vi "Override maxSensorNum (O).vi"(8 "Error In":errorcluster, 10 "Max. number of sensors":u8 max=64, 11 "VISA resource name in":refnum<visa-resource-name>) -> (0 "Error out":errorcluster, 1 "ACK":bool, 2 "L_data":u16, 3 "VISA resource name out":refnum<visa-resource-name>)   [LabVIEW 2015]
uses:
  Ctls/Cmd str.ctl
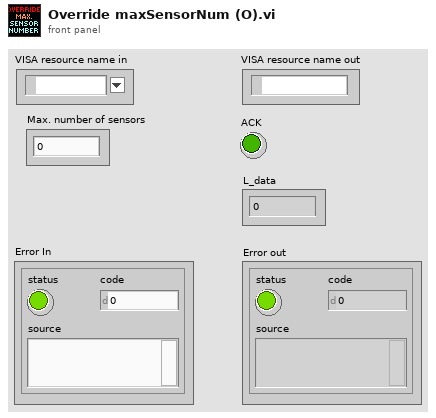
[diagram p1: front panel]
types:
  T1 = typedef "Cmd str.ctl" = string
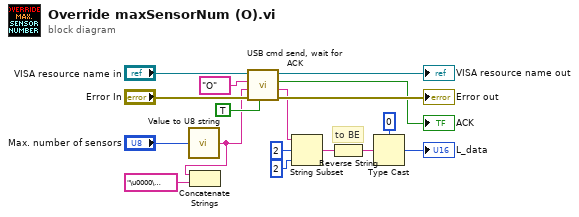
[diagram p0: block diagram]
diagram:
  # "to BE"
  n1 = call "Value to U8 string.vi"("Value"="Max. number of sensors") -> ("U8 str"=w9:string)
  n2 = Concatenate Strings(w9, "\u0000\u0000\u0000" ("string")) -> ()  [unwired: 1 out]
  n3 = call "USB cmd send, wait for ACK.vi"("Wait for ACK?"=TRUE, "Error In"="Error In", "4 byte config str"=w9, "Cmd"=T1 "O", "VISA resource name in"="VISA resource name in") -> ("Error out"=→"Error out":errorcluster, "Return msg"=w1:string, "ACK ok"=→"ACK":bool, "VISA resource name out"=→"VISA resource name out":refnum<visa-resource-name>)  [unwired: 1 in]
  n4 = String Subset(string=w1, offset (0)=2, length (rest)=2 ("length (rest)")) -> (substring=w5:string)
  n5 = Reverse String(1:w5) -> (0:w2:string)
  n6 = Type Cast(type=u16 0 ("offset (0)"), x=w2) -> (*(type *) &x=→"L_data":u16)
